vi "R5Master.vi"(6 "LabVIEW Web Service":refnum<class "Web Service.lvclass">=refnum) -> ()   [LabVIEW 2016]
uses:
  <vilib>/wsapi/Web Service.lvclass
  Controls/pH_SetParams Standard.ctl
  R5Controls/R5SBR_SetParams.ctl
  <vilib>/Platform/TimedLoop/XDataNode/timing_clust.ctl
  <vilib>/Platform/TimedLoop/XDataNode/nitl_modes.ctl
  <vilib>/Platform/TimedLoop/XDataNode/wakeup.ctl
  <vilib>/Platform/TimedLoop/XDataNode/loadnilvce.vi
  <vilib>/Platform/TimedLoop/XDataNode/XDataNode.xnode
  <vilib>/Platform/TimedLoop/XDataNode/XDNodeRunTimeDep.lvlib
panel:
  in  "NH4 Pump":bool
  in  "R5 NH4_FeedParams":T1
  in  "R5SBR_SetParams":T2=[{"Phase"="Feed", "Time, min"=2.0, "SBR_Manual"={"Influent Pump"=TRUE, "Effluent Pump"=TRUE}}, {"Phase"="Batch", "Time, min"=58.0, "SBR_Manual"={"Influent Pump"=FALSE, "Effluent Pump"=FALSE}}]
  out "Probes":cluster{"Value":dbl, "Value":dbl}(graph)={"Value"=7.553744624219178, "Value"=7.151824862435147}
  in  "R5SBRManual":cluster{"Media Pump":bool, "Effluent Pump":bool}
  out "error out":errorcluster
  out "error out (DATA COLLECT)":errorcluster
  out "error out (SBR)":errorcluster
  in  "R5 SBR_Switch":bool
  in  "R5DOManual":cluster{"Air MFC":dbl, "N2 MFC":dbl} {"Air MFC" scale=0.0..500.0; "N2 MFC" scale=0.0..500.0}
  in  "R5 DO_Switch":bool
  out "R5DO":cluster{"Signal":dbl, "Value":dbl}={"Signal"=0.009325505850500406, "Value"=7.5541599264321775}
  in  "R5 pH_Switch":bool
  in  "R5 pH_SetParams":T3={"Set Point"=7.5, "Tolerance"=0.1, "Pump Time On, secs"=6.0}
  in  "R5pH_Manual":cluster{"Acid Pump":bool, "Base Pump":bool}
  out "pH":cluster{"Signal":dbl, "Value":dbl}={"Signal"=0.011346734125719843, "Value"=7.151648980100406}
  out "Timestamp":string="05/02/2018 13:19:24.640"
  out "Status":string="Off"
  out "Cycle Time Elapsed":dbl
  out "Phase Time Elapsed":dbl
  # "Use the web service input terminal to call the VIs on the Service subpalette of the Web Services palette. Do not remove it from the connector pane unless you don't need access to the palette."
  # "Any additional terminals added to the connector pane of a startup VI will be ignored."
  # "DO Control"
  # "SBR Control"
  # "pH Control"
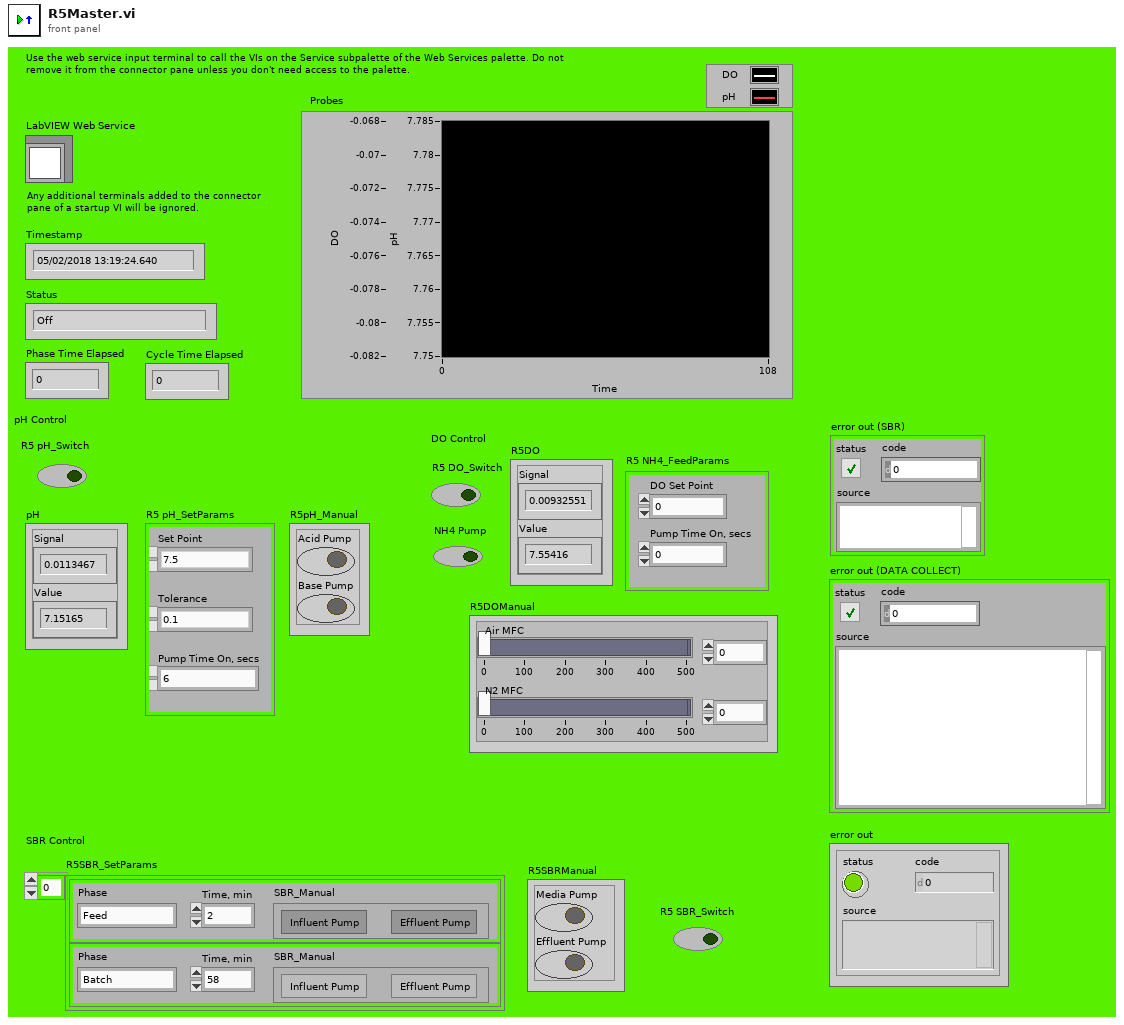
[diagram p1: front panel]
types:
  T1 = cluster{"DO Set Point":dbl, "Pump Time On, secs":dbl}
  T2 = typedef "R5SBR_SetParams.ctl" = cluster{"Phase":string, "Time, min":dbl, "SBR_Manual":cluster{"Influent Pump":bool, "Effluent Pump":bool}}[]
  T3 = typedef "pH_SetParams Standard.ctl" = cluster{"Set Point":dbl, "Tolerance":dbl, "Pump Time On, secs":dbl}
  T4 = typedef "XDNodeRunTimeDep.lvlib/timing_clust.ctl" = cluster{"Expected End [f-1]":u64, "Actual End [f-1]":u64, "Finished Late? [f-1]":bool, "Expected End [i-1]":u64, "Actual End [i-1]":u64, "Finished Late? [i-1]":bool, "Expected Start [i]":u64, "Actual Start [i]":u64, "Expected Start [f]":u64, "Actual Start [f]":u64, "Source Name":string, "Structure Name":string, "Period":i64, "Deadline":i64, "Offset":i64, "Start":i64, "Priority":i32, "Timeout":i32, "Mode":T5, "Wakeup Reason":T6, "Error":errorcluster, "Source Type":string, "Secondary Source Type":string, "Global End Time":u64, "Global Start Time":u64, "Frame Duration":u64, "Iteration Duration":u64, "Assigned CPU":i32, "I/O Scan Engine Mode":u32}
  T5 = typedef "XDNodeRunTimeDep.lvlib/nitl_modes.ctl" = enum32{"No Change", "Process missed periods, maintain original phase", "Discard missed periods, maintain original phase", "Process missed periods, ignore original phase", "Discard missed periods, ignore original phase"}
  T6 = typedef "XDNodeRunTimeDep.lvlib/wakeup.ctl" = enum32{"Normal", "Aborted", "Asynchronous wakeup", "Timing source error", "Timed loop error", "Timeout"}
  T7 = enum8{"Enabled", "Disabled", "Disabled and Grayed Out"}
  T8 = cluster{"Influent Pump":bool, "Effluent Pump":bool}
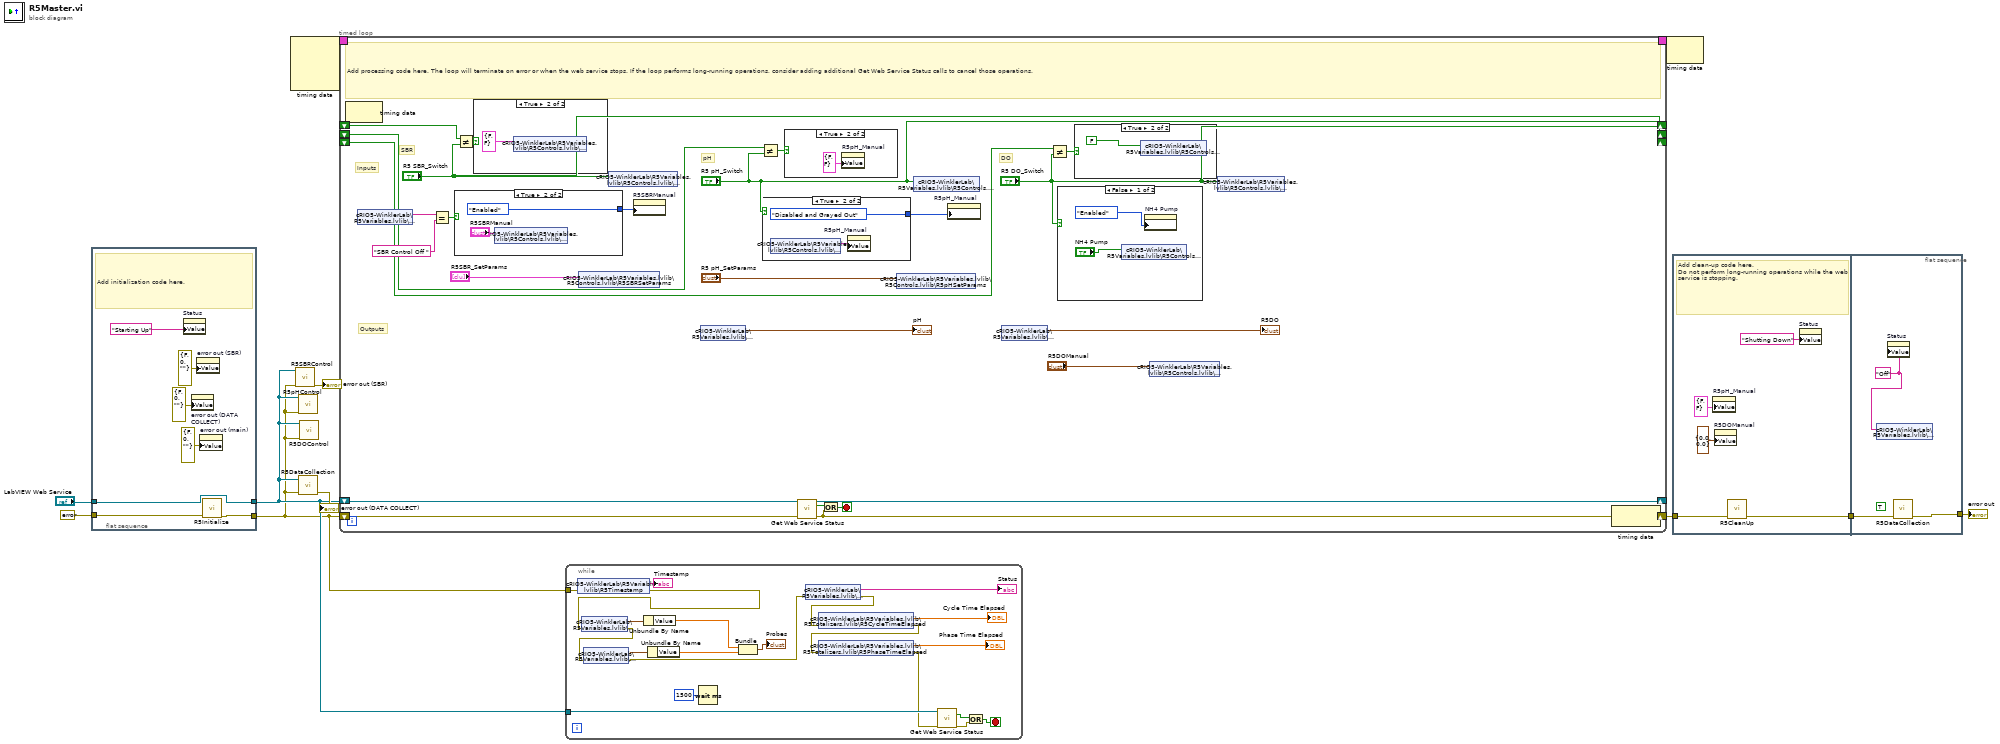
[diagram p0: block diagram]
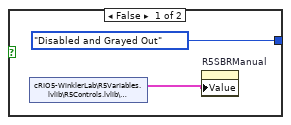
[diagram p5: hidden frame]
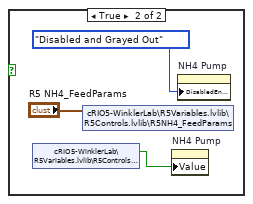
[diagram p6: hidden frame]
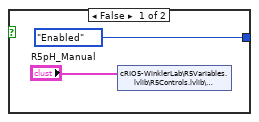
[diagram p7: hidden frame]
diagram:
  n1 = flat-sequence {
    tunnel: "LabVIEW Web Service" -> [w18]
    tunnel: errorcluster {"status"=FALSE, "code"=0, "source"=""} ("error constant") -> [w12]
    tunnel: [w13] -> w1
    tunnel: [w18] -> w2
    frame #0 {
      # "Add initialization code here."
      n2 = property on="Status" class="Str"("Value"="Starting Up" ("Status")) -> ()  [unwired: 2 in, 2 out]
      n3 = property on="error out (DATA COLLECT)" class="Clust (strict)"("Value"=errorcluster {"status"=FALSE, "code"=0, "source"=""} ("error out (DATA COLLECT)")) -> ()  [unwired: 2 in, 2 out]
      n4 = property on="error out (SBR)" class="Clust (strict)"("Value"=errorcluster {"status"=FALSE, "code"=0, "source"=""} ("error out (SBR)")) -> ()  [unwired: 2 in, 2 out]
      n5 = property on="error out (main)" class="Clust (strict)"("Value"=errorcluster {"status"=FALSE, "code"=0, "source"=""} ("error out")) -> ()  [unwired: 2 in, 2 out]
      n6 = call "R5Initialize.vi"("error in (no error)"=w12) -> ("error out"=w13:errorcluster)  [unwired: 10 in]
    }
  }
  n7 = node-c288() -> (w8:T4)  [unwired: 4 in]
  n8 = call "R5SBRControl.vi"("error constant"=w1, "LabVIEW Web Service"=w2) -> ("error out"=→"error out (SBR)":errorcluster)  [unwired: 9 in]
  n9 = call "R5pHControl.vi"("error constant"=w1, "LabVIEW Web Service"=w2) -> ()  [unwired: 10 in]
  n10 = call "R5DataCollection.vi"("error constant"=w1, "LabVIEW Web Service"=w2) -> ("error out"=→"error out (DATA COLLECT)":errorcluster)  [unwired: 9 in]
  n11 = call "R5DOControl.vi"("error constant"=w1, "LabVIEW Web Service"=w2) -> ()  [unwired: 10 in]
  n12 = timed-loop {
    shift-right: [w41] -> w9
    shift-left: w1 -> [w40]
    shift-right: [w38] -> _
    shift-left: w2 -> [w38]
    timing: w8 -> [_]
    timing-out: [_] -> w7
    shift-right: ["R5 SBR_Switch"] -> _
    shift-left: _ -> [w29]
    shift-right: ["R5 pH_Switch"] -> _
    shift-left: _ -> [w35]
    shift-right: ["R5 DO_Switch"] -> _
    shift-left: _ -> [w33]
    stop <- w39 stop-if-true
    # "DO"
    # "pH"
    # "Outputs"
    # "Inputs"
    # "SBR"
    # "Add processing code here. The loop will terminate on error or when the web service stops. If the loop performs long-running operations, consider adding additional Get Web Service Status calls to cancel those operations."
    n13 = node-c288() -> ()  [unwired: 1 in, 1 out]
    n14 = shared-variable "cRIO5-WinklerLab\\R5Variables.lvlib\\R5Status"() -> (w28:string)  [unwired: 1 in, 1 out]
    n15 = Equal?(x=w28, y="SBR Control Off " ("string")) -> (x = y?=w30:bool)
    n16 = case shown="True" w30 {
      tunnel: [T7."Disabled and Grayed Out" ("Disabled") T7."Enabled" ("Disabled")] -> w22
      frame False {
        n17 = shared-variable "cRIO5-WinklerLab\\R5Variables.lvlib\\R5Controls.lvlib\\R5SBRManual"() -> (w46:T8)  [unwired: 1 in, 1 out]
        n18 = property on="R5SBRManual" class="Clust (strict)"("Value"=w46) -> ()  [unwired: 2 in, 2 out]
      }
      frame True {
        n19 = shared-variable "cRIO5-WinklerLab\\R5Variables.lvlib\\R5Controls.lvlib\\R5SBRManual"("R5SBRManual") -> ()  [unwired: 1 in, 1 out]
      }
    }
    n20 = Not Equal?(x=w29, y="R5 SBR_Switch") -> (x != y?=w36:bool)
    n21 = case shown="True" w36 {
      frame False {
      }
      frame True {
        n22 = shared-variable "cRIO5-WinklerLab\\R5Variables.lvlib\\R5Controls.lvlib\\R5SBRManual"(cluster{"Media Pump":bool, "Effluent Pump":bool} {"Media Pump"=FALSE, "Effluent Pump"=FALSE} ("R5SBRManual")) -> ()  [unwired: 1 in, 1 out]
      }
    }
    n23 = shared-variable "cRIO5-WinklerLab\\R5Variables.lvlib\\R5Controls.lvlib\\R5SBRSetParams"("R5SBR_SetParams") -> ()  [unwired: 1 in, 1 out]
    n24 = shared-variable "cRIO5-WinklerLab\\R5Variables.lvlib\\R5Controls.lvlib\\R5SBRSwitch"("R5 SBR_Switch") -> ()  [unwired: 1 in, 1 out]
    n25 = property on="R5SBRManual" class="Clust (strict)"("DisabledEnum"=w22) -> ()  [unwired: 2 in, 2 out]
    n26 = shared-variable "cRIO5-WinklerLab\\R5Variables.lvlib\\R5Signals.lvlib\\R5pH"() -> (→"pH":cluster{"Signal":dbl, "Value":dbl})  [unwired: 1 in, 1 out]
    n27 = Not Equal?(x=w35, y="R5 pH_Switch") -> (x != y?=w34:bool)
    n28 = case shown="True" "R5 pH_Switch" {
      tunnel: [T7."Enabled" ("Disabled") T7."Disabled and Grayed Out" ("Disabled")] -> w37
      frame False {
        n29 = shared-variable "cRIO5-WinklerLab\\R5Variables.lvlib\\R5Controls.lvlib\\R5pHManual"("R5pH_Manual") -> ()  [unwired: 1 in, 1 out]
      }
      frame True {
        n30 = shared-variable "cRIO5-WinklerLab\\R5Variables.lvlib\\R5Controls.lvlib\\R5pHManual"() -> (w57:cluster{"Acid Pump":bool, "Base Pump":bool})  [unwired: 1 in, 1 out]
        n31 = property on="R5pH_Manual" class="Clust (strict)"("Value"=w57) -> ()  [unwired: 2 in, 2 out]
      }
    }
    n32 = case shown="True" w34 {
      frame False {
      }
      frame True {
        n33 = property on="R5pH_Manual" class="Clust (strict)"("Value"=cluster{"Acid Pump":bool, "Base Pump":bool} {"Acid Pump"=FALSE, "Base Pump"=FALSE} ("R1pH_Manual")) -> ()  [unwired: 2 in, 2 out]
      }
    }
    n34 = call <vilib>:"Get Web Service Status.vi"("LabVIEW Web Service"=w38, "error in (no error)"=w40) -> ("service stopping?"=w42:bool, "error out"=w41:errorcluster)  [unwired: 11 in, 1 out]
    n35 = Or(x=w42, y=w41) -> (x .or. y?=w39:bool)
    n36 = shared-variable "cRIO5-WinklerLab\\R5Variables.lvlib\\R5Controls.lvlib\\R5pHSetParams"("R5 pH_SetParams") -> ()  [unwired: 1 in, 1 out]
    n37 = shared-variable "cRIO5-WinklerLab\\R5Variables.lvlib\\R5Controls.lvlib\\R5pHSwitch"("R5 pH_Switch") -> ()  [unwired: 1 in, 1 out]
    n38 = property on="R5pH_Manual" class="Clust (strict)"("DisabledEnum"=w37) -> ()  [unwired: 2 in, 2 out]
    n39 = shared-variable "cRIO5-WinklerLab\\R5Variables.lvlib\\R5Signals.lvlib\\R5DO"() -> (→"R5DO":cluster{"Signal":dbl, "Value":dbl})  [unwired: 1 in, 1 out]
    n40 = Not Equal?(x=w33, y="R5 DO_Switch") -> (x != y?=w32:bool)
    n41 = case shown="False" "R5 DO_Switch" {
      frame False {
        n42 = shared-variable "cRIO5-WinklerLab\\R5Variables.lvlib\\R5Controls.lvlib\\R5NH4Feed"("NH4 Pump") -> ()  [unwired: 1 in, 1 out]
        n43 = property on="NH4 Pump" class="Bool (strict)"("DisabledEnum"=T7."Enabled" ("Disabled")) -> ()  [unwired: 2 in, 2 out]
      }
      frame True {
        n44 = shared-variable "cRIO5-WinklerLab\\R5Variables.lvlib\\R5Controls.lvlib\\R5NH4Feed"() -> (w53:bool)  [unwired: 1 in, 1 out]
        n45 = shared-variable "cRIO5-WinklerLab\\R5Variables.lvlib\\R5Controls.lvlib\\R5NH4_FeedParams"("R5 NH4_FeedParams") -> ()  [unwired: 1 in, 1 out]
        n46 = property on="NH4 Pump" class="Bool (strict)"("Value"=w53) -> ()  [unwired: 2 in, 2 out]
        n47 = property on="NH4 Pump" class="Bool (strict)"("DisabledEnum"=T7."Disabled and Grayed Out" ("Disabled")) -> ()  [unwired: 2 in, 2 out]
      }
    }
    n48 = case shown="True" w32 {
      frame False {
      }
      frame True {
        n49 = shared-variable "cRIO5-WinklerLab\\R5Variables.lvlib\\R5Controls.lvlib\\R5NH4Feed"(FALSE) -> ()  [unwired: 1 in, 1 out]
      }
    }
    n50 = shared-variable "cRIO5-WinklerLab\\R5Variables.lvlib\\R5Controls.lvlib\\R5DOManual"("R5DOManual") -> ()  [unwired: 1 in, 1 out]
    n51 = shared-variable "cRIO5-WinklerLab\\R5Variables.lvlib\\R5Controls.lvlib\\R5DOSwitch"("R5 DO_Switch") -> ()  [unwired: 1 in, 1 out]
    n52 = node-c288() -> ()  [unwired: 1 in, 1 out]
  }
  n53 = while {
    tunnel: w2 -> [w80]
    tunnel: w1 -> [w74]
    stop <- w77 stop-if-true
    n54 = shared-variable "cRIO5-WinklerLab\\R5Variables.lvlib\\R5Timestamp"(error in=w74) -> (→"Timestamp":string, error out=w67:errorcluster)
    n55 = shared-variable "cRIO5-WinklerLab\\R5Variables.lvlib\\R5Signals.lvlib\\R5DO"(error in=w67) -> (w69:cluster{"Signal":dbl, "Value":dbl}, error out=w68:errorcluster)
    n56 = shared-variable "cRIO5-WinklerLab\\R5Variables.lvlib\\R5Signals.lvlib\\R5pH"(error in=w68) -> (w71:cluster{"Signal":dbl, "Value":dbl}, error out=w70:errorcluster)
    n57 = Unbundle By Name(w69) -> ("Value"=w81:dbl)
    n58 = Unbundle By Name(w71) -> ("Value"=w75:dbl)
    n59 = Wait (ms)(milliseconds to wait=u32 1500) -> ()  [unwired: 1 out]
    n60 = Bundle("Value"=w81, "Value"=w75) -> (→"Probes":cluster{"Value":dbl, "Value":dbl})  [unwired: 1 in]
    n61 = shared-variable "cRIO5-WinklerLab\\R5Variables.lvlib\\R5Status"(error in=w70) -> (→"Status":string, error out=w66:errorcluster)
    n62 = shared-variable "cRIO5-WinklerLab\\R5Variables.lvlib\\R5Totalizers.lvlib\\R5CycleTimeElapsed"(error in=w66) -> (→"Cycle Time Elapsed":dbl, error out=w62:errorcluster)
    n63 = shared-variable "cRIO5-WinklerLab\\R5Variables.lvlib\\R5Totalizers.lvlib\\R5PhaseTimeElapsed"(error in=w62) -> (→"Phase Time Elapsed":dbl, error out=w63:errorcluster)
    n64 = call <vilib>:"Get Web Service Status.vi"("LabVIEW Web Service"=w80, "error in (no error)"=w63) -> ("service stopping?"=w79:bool, "error out"=w78:errorcluster)  [unwired: 11 in, 1 out]
    n65 = Or(x=w79, y=w78) -> (x .or. y?=w77:bool)
  }
  n66 = node-c288(w7) -> ()  [unwired: 1 out]
  n67 = flat-sequence {
    tunnel: w9 -> [w82]
    tunnel: [w83] -> w6
    tunnel: w6 -> [w88]
    tunnel: [w87] -> w5
    frame #0 {
      # "Add clean-up code here.\nDo not perform long-running operations while the web service is stopping."
      n68 = property on="R5pH_Manual" class="Clust (strict)"("Value"=cluster{"Acid Pump":bool, "Base Pump":bool} {"Acid Pump"=FALSE, "Base Pump"=FALSE} ("R1pH_Manual")) -> ()  [unwired: 2 in, 2 out]
      n69 = property on="R5DOManual" class="Clust (strict)"("Value"=cluster{"Air MFC":dbl, "N2 MFC":dbl} {"Air MFC"=0.0, "N2 MFC"=0.0} ("R1DOManual")) -> ()  [unwired: 2 in, 2 out]
      n70 = call "R5CleanUp.vi"("error in (no error)"=w82) -> ("error out"=w83:errorcluster)  [unwired: 10 in]
      n71 = property on="Status" class="Str"("Value"="Shutting Down" ("Status")) -> ()  [unwired: 2 in, 2 out]
    }
    frame #1 {
      w89 = "Off" ("Status")
      (unwired) TRUE ("Write Once")
      n72 = shared-variable "cRIO5-WinklerLab\\R5Variables.lvlib\\R5Status"(w89) -> ()  [unwired: 1 in, 1 out]
      n73 = property on="Status" class="Str"("Value"=w89) -> ()  [unwired: 2 in, 2 out]
      n74 = call "R5DataCollection.vi"("error constant"=w88) -> ("error out"=w87:errorcluster)  [unwired: 10 in]
    }
  }
  "error out" <- w5
